vi "2013_01_03 Flow Motor.vi"(0 "Motor Typedef":T2={"Fail"=FALSE, "RPM"=0, "Motor"=enum."Maxon EC6 6V", "ESC"=enum."Phoenix 10", "Supply (V)"=0.0, "Elapsed Time"=0.0, "Counter"=0.0, "Torque (mNm)"=0.0, "Electrical Power (W)"=0.0, "Motor Efficiency"=0.0, "Mechanical Power (W)"=0.0, "Supply Power (W)"=0.0, "ESC Efficiency"=0.0, "PWM"=0, "Direction"=enum."Push"} {"PWM" min=0 max=100 step=1 scale=0.0..100.0; "ESC Efficiency" format="%#_3g%%"; "Supply Power (W)" format="%.3g"; "Mechanical Power (W)" format="%.3g"; "Motor Efficiency" format="%#_3g%%"; "Electrical Power (W)" format="%.3g"; "Torque (mNm)" format="%.3g"; "Elapsed Time" format="%<%H:%M:%S>t"; "Supply (V)" format="%.2f"; "RPM" scale=0.0..60000.0}, 1 "Motor Typedef 2":T2={"Fail"=FALSE, "RPM"=0, "Motor"=enum."Maxon EC6 6V", "ESC"=enum."Phoenix 10", "Supply (V)"=0.0, "Elapsed Time"=0.0, "Counter"=0.0, "Torque (mNm)"=0.0, "Electrical Power (W)"=0.0, "Motor Efficiency"=0.0, "Mechanical Power (W)"=0.0, "Supply Power (W)"=0.0, "ESC Efficiency"=0.0, "PWM"=0, "Direction"=enum."Push"} {"PWM" min=0 max=100 step=1 scale=0.0..100.0; "ESC Efficiency" format="%#_3g%%"; "Supply Power (W)" format="%.3g"; "Mechanical Power (W)" format="%.3g"; "Motor Efficiency" format="%#_3g%%"; "Electrical Power (W)" format="%.3g"; "Torque (mNm)" format="%.3g"; "Elapsed Time" format="%<%H:%M:%S>t"; "Supply (V)" format="%.2f"; "RPM" scale=0.0..60000.0}, 2 "Capture":bool, 5 "File Path":path, 6 "Zero":bool, 7 "Save":bool, 8 "Flow in":T1 {"Thermometer" scale=15.0..50.0; "Pressure Up (mmHg)" format="%#.1g"; "Pressure Down (mmHg)" format="%#.1g"; "Zero Up" format="%.2f"; "Hydraulic Power" scale=0.0..0.1 scale format="%#.2f"; "Flow" scale=0.0..8.0 scale format="%#.2f"; "Pressure Difference" scale=0.0..10.0 scale format="%#.2f"}, 9 "data":waveform(dbl)[](array[waveform]), 11 "File ID and Serial #s":string, 12 "DAQmx Task Name":refnum<k21>, 13 "Clear":bool, 14 "Comment":string) -> (3 "Motor Typedef Out 2":T2={"Fail"=FALSE, "RPM"=0, "Motor"=enum."Maxon EC6 6V", "ESC"=enum."Phoenix 10", "Supply (V)"=0.0, "Elapsed Time"=0.0, "Counter"=0.0, "Torque (mNm)"=0.0, "Electrical Power (W)"=0.0, "Motor Efficiency"=0.0, "Mechanical Power (W)"=0.0, "Supply Power (W)"=0.0, "ESC Efficiency"=0.0, "PWM"=0, "Direction"=enum."Push"} {"PWM" min=0 max=100 step=1 scale=0.0..100.0; "ESC Efficiency" format="%#_3g%%"; "Supply Power (W)" format="%.3g"; "Mechanical Power (W)" format="%.3g"; "Motor Efficiency" format="%#_3g%%"; "Electrical Power (W)" format="%.3g"; "Torque (mNm)" format="%.3g"; "Elapsed Time" format="%<%H:%M:%S>t"; "Supply (V)" format="%.2f"; "RPM" scale=0.0..60000.0}, 4 "Motor Typedef Out":T2={"Fail"=FALSE, "RPM"=0, "Motor"=enum."Maxon EC6 6V", "ESC"=enum."Phoenix 10", "Supply (V)"=0.0, "Elapsed Time"=0.0, "Counter"=0.0, "Torque (mNm)"=0.0, "Electrical Power (W)"=0.0, "Motor Efficiency"=0.0, "Mechanical Power (W)"=0.0, "Supply Power (W)"=0.0, "ESC Efficiency"=0.0, "PWM"=0, "Direction"=enum."Push"} {"PWM" min=0 max=100 step=1 scale=0.0..100.0; "ESC Efficiency" format="%#_3g%%"; "Supply Power (W)" format="%.3g"; "Mechanical Power (W)" format="%.3g"; "Motor Efficiency" format="%#_3g%%"; "Electrical Power (W)" format="%.3g"; "Torque (mNm)" format="%.3g"; "Elapsed Time" format="%<%H:%M:%S>t"; "Supply (V)" format="%.2f"; "RPM" scale=0.0..60000.0}, 10 "Flow and P out":T1 {"Thermometer" scale=15.0..50.0; "Pressure Up (mmHg)" format="%#.1g"; "Pressure Down (mmHg)" format="%#.1g"; "Zero Up" format="%.2f"; "Hydraulic Power" scale=0.0..0.1 scale format="%#.2f"; "Flow" scale=0.0..8.0 scale format="%#.2f"; "Pressure Difference" scale=0.0..10.0 scale format="%#.2f"}, 15 "Final Out":dynamicdata(graph))   [LabVIEW 2013]
uses:
  Flow Type Def.ctl
  flow and pressure.ctl
  <vilib>/measure/madcrms.llb/Basic Averaged DC-RMS for 1 Chan.vi
  <vilib>/express/express shared/transition.llb/Dynamic To Waveform Array.vi
  <vilib>/express/express signal manip/GetorSetDDTAttributes/Set DDT Attributes/SetT0.vi
  <vilib>/express/express shared/transition.llb/Waveform Array To Dynamic.vi
  <vilib>/express/express signal manip/GetorSetDDTAttributes/Set DDT Attributes/Set DDT Properties.xnode
  <vilib>/measure/NI_MAPro.lvlib
panel:
  in  "Motor 2 Enable":bool
  in  "error in (no error)":errorcluster
  out "error out":errorcluster
  out "Saving Data":bool
  # "Stopped"
  # "Stopped"
  # "Stopped"
  # "Stopped"
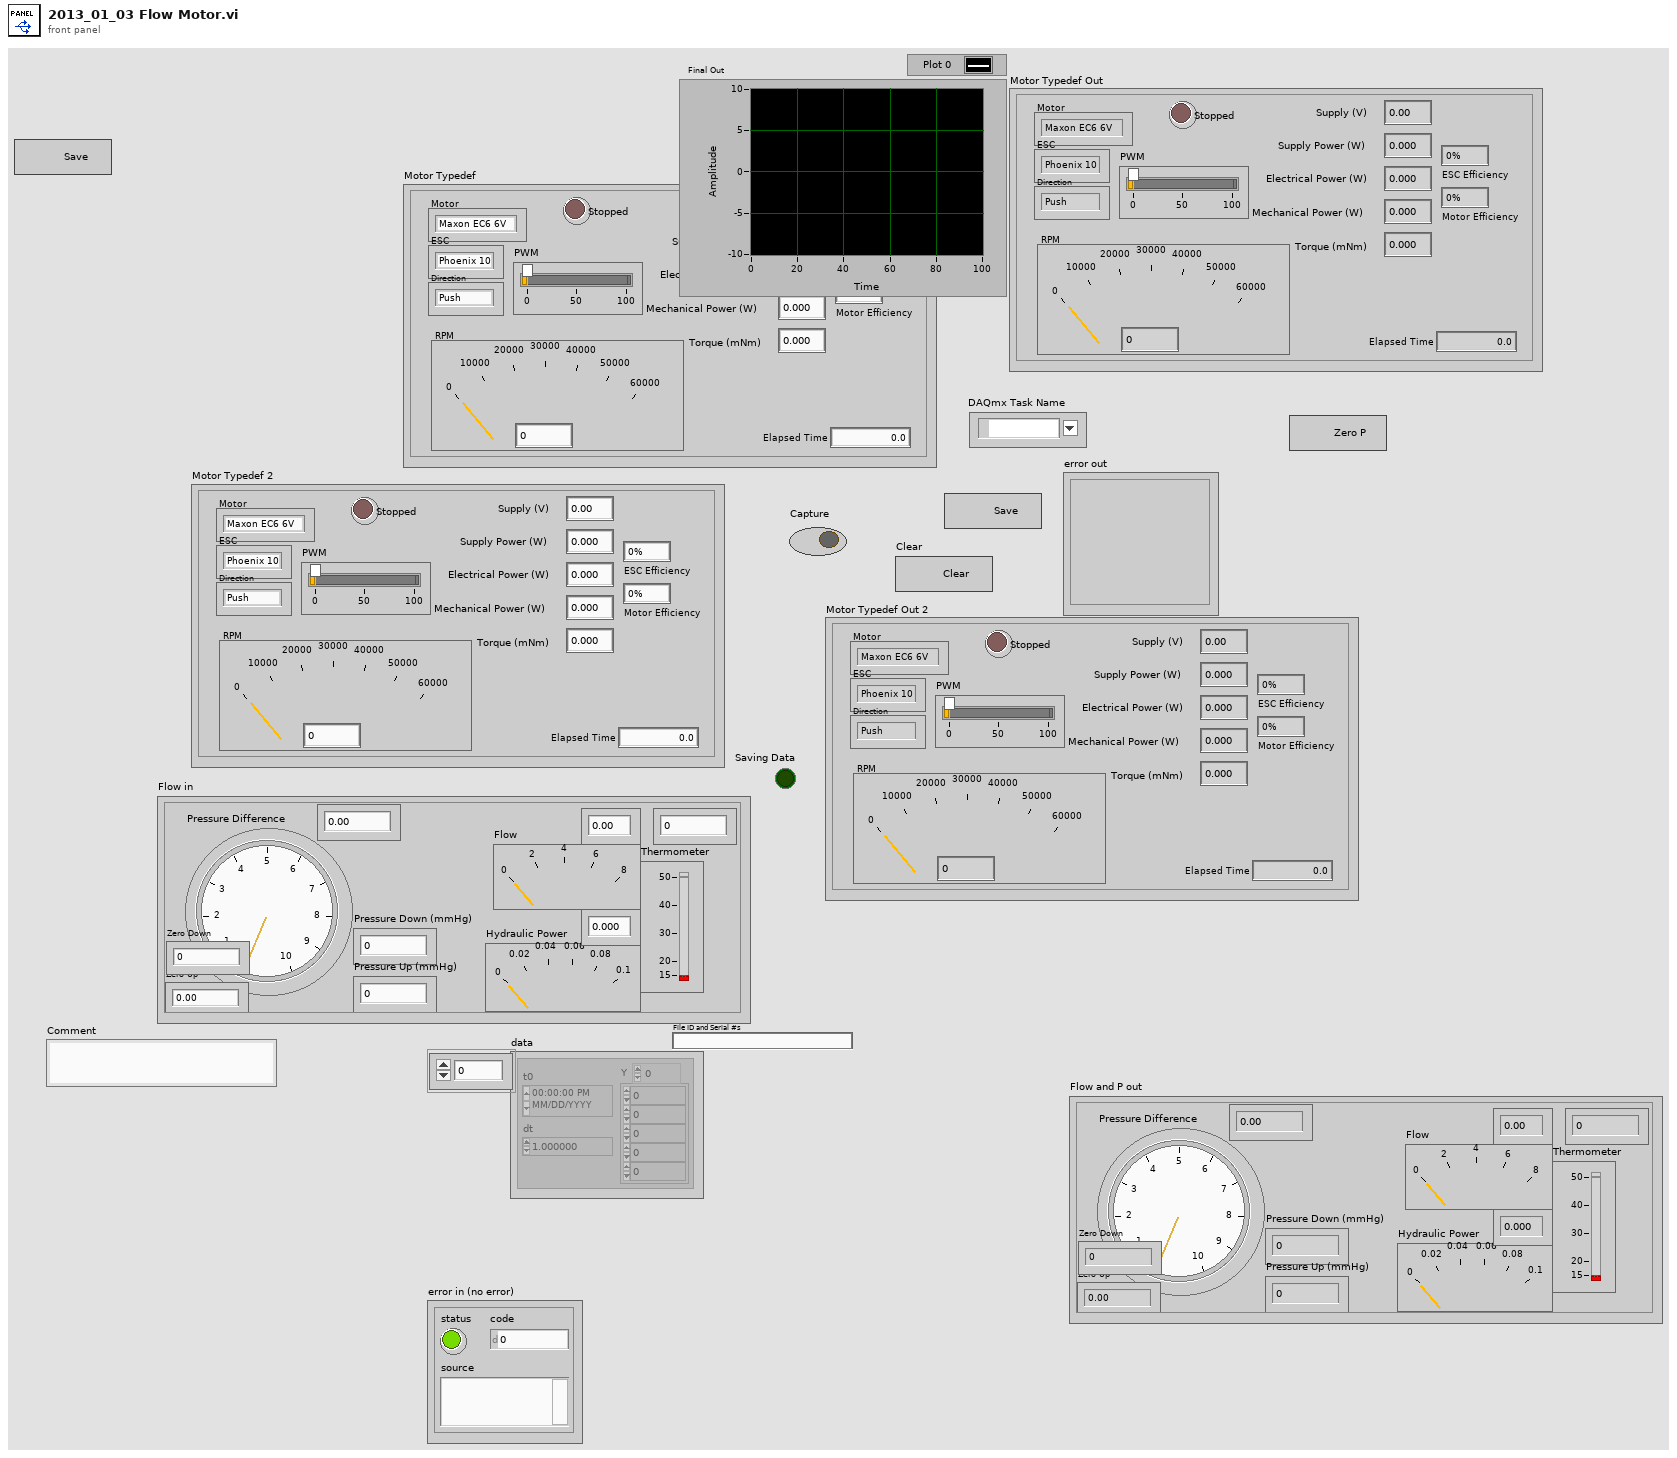
[diagram p1: front panel]
types:
  T1 = typedef "flow and pressure.ctl" = cluster{"Pressure Difference":dbl, "Flow":dbl, "Hydraulic Power":dbl, "Zero Up":dbl, "Pressure Down (mmHg)":dbl, "Pressure Up (mmHg)":dbl, "Zero Down":dbl, "Thermometer":dbl}
  T2 = typedef "Flow Type Def.ctl" = cluster{"Fail":bool, "RPM":u64, "Motor":enum16{"", "Maxon EC6 6V", "Maxon EC4 6V", "FH 0620 6V", "FH 0620 12V", "FH 0427"}, "ESC":enum16{"Phoenix 10", "Maxon", "FH 1801"}, "Supply (V)":dbl, "Elapsed Time":dbl, "Counter":dbl, "Torque (mNm)":dbl, "Electrical Power (W)":dbl, "Motor Efficiency":dbl, "Mechanical Power (W)":dbl, "Supply Power (W)":dbl, "ESC Efficiency":dbl, "PWM":i32, "Direction":enum16{"Push", "Pull"}}
  T3 = enum16{"", "Maxon EC6 6V", "Maxon EC4 6V", "FH 0620 6V", "FH 0620 12V", "FH 0427"}
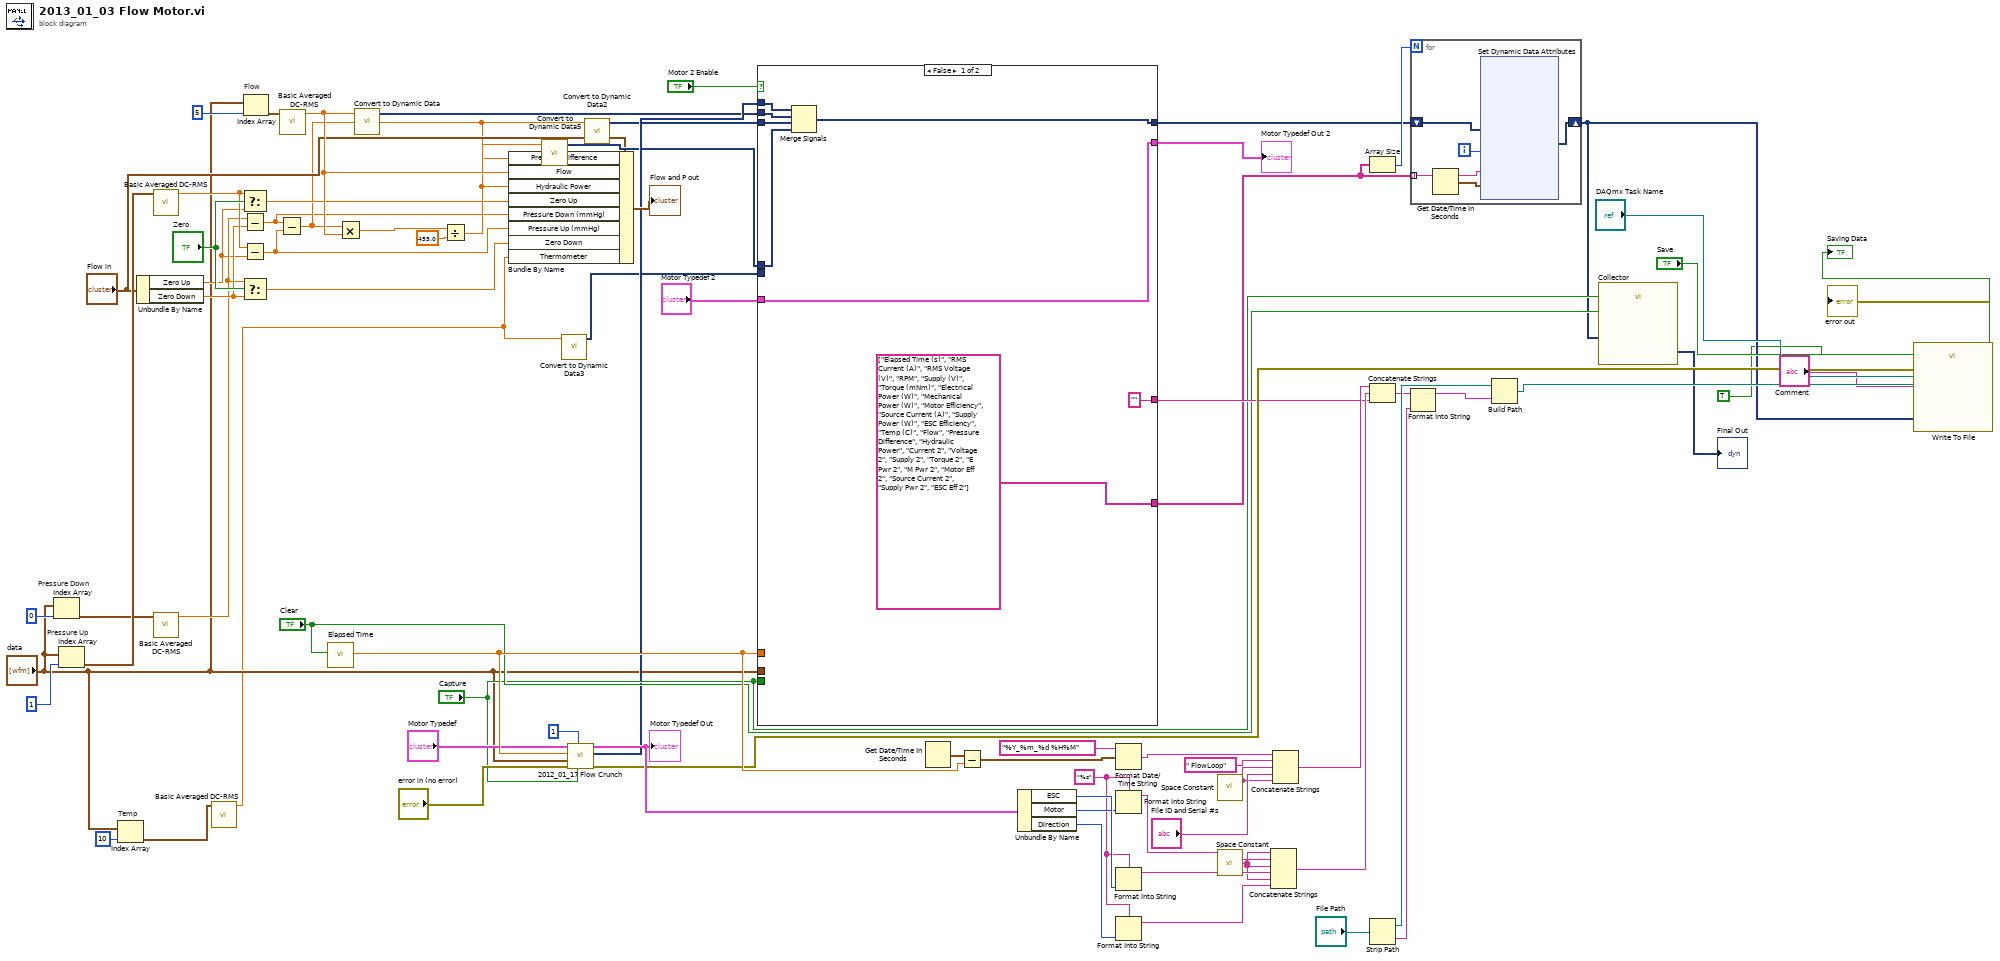
[diagram p0: block diagram]
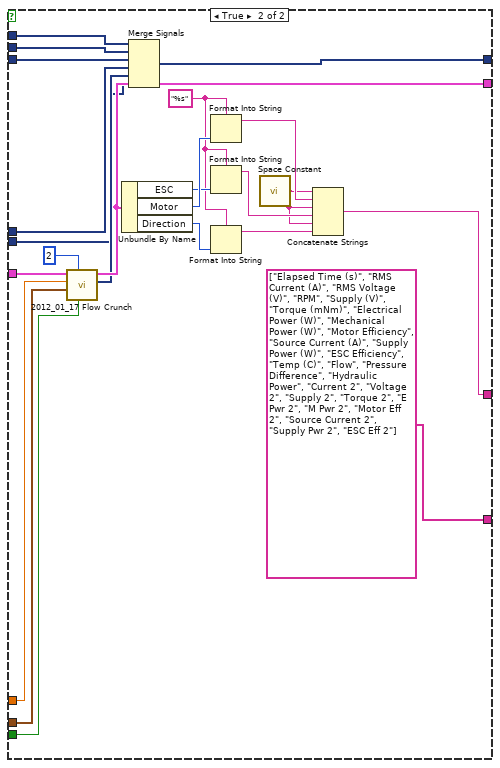
[diagram p2: hidden frame]
diagram:
  w30 = "%s" ("format string")
  n1 = Index Array "Pressure Down"(array="data", index=0) -> (element=w46:waveform(dbl))
  n2 = Index Array "Pressure Up"(array="data", index=1) -> (element=w47:waveform(dbl))
  n3 = Index Array "Temp"(array="data", index=10) -> (element=w5:waveform(dbl))
  n4 = Unbundle By Name("Flow in") -> ("Zero Up"=w10:dbl, "Zero Down"=w13:dbl)
  n5 = call-poly <vilib>:"Basic Averaged DC-RMS.vi"("signal in"=w47) -> ("DC value"=w14:dbl)  [unwired: 7 in, 3 out]
  n6 = call-poly <vilib>:"Basic Averaged DC-RMS.vi"("signal in"=w46) -> ("DC value"=w12:dbl)  [unwired: 7 in, 3 out]
  n7 = call-poly <vilib>:"Basic Averaged DC-RMS.vi"("signal in"=w5) -> ("DC value"=w4:dbl)  [unwired: 7 in, 3 out]
  n8 = Select(t=w14, s="Zero", f=w10) -> (s? t:f=w19:dbl)
  n9 = Subtract(x=w12, y=w13) -> (x-y=w9:dbl)
  n10 = Subtract(x=w14, y=w10) -> (x-y=w8:dbl)
  n11 = Select(t=w12, s="Zero", f=w13) -> (s? t:f=w15:dbl)
  n12 = Index Array "Flow"(array="data", index=5) -> (element=w48:waveform(dbl))
  n13 = Subtract(x=w9, y=w8) -> (x-y=w11:dbl)
  n14 = call-poly <vilib>:"Basic Averaged DC-RMS.vi"("signal in"=w48) -> ("DC value"=w41:dbl)  [unwired: 7 in, 3 out]
  n15 = call "Elapsed Time"("Reset"="Clear") -> ("Elapsed Time (s)"=w75:dbl)  [unwired: 11 in, 7 out]
  n16 = Multiply(x=w11, y=w41) -> (x*y=w40:dbl)
  n17 = call "Convert to Dynamic Data"("Double"=w41) -> ("Dynamic Data Type"=w24:dynamicdata)  [unwired: 3 in]
  n18 = Divide(x=w40, y=455.0) -> (x/y=w38:dbl)
  n19 = Bundle By Name(cluster="Flow in", "Pressure Difference"=w11, "Flow"=w41, "Hydraulic Power"=w38, "Zero Up"=w19, "Pressure Down (mmHg)"=w9, "Pressure Up (mmHg)"=w8, "Zero Down"=w15, "Thermometer"=w4) -> (→"Flow and P out":T1)
  n20 = call "Convert to Dynamic Data5"("Double"=w38) -> ("Dynamic Data Type"=w23:dynamicdata)  [unwired: 3 in]
  n21 = call "Convert to Dynamic Data3"("Double"=w4) -> ("Dynamic Data Type"=w3:dynamicdata)  [unwired: 3 in]
  n22 = call "2012_01_17 Flow Crunch.vi"("Capture"="Capture", "Motor #"=1, "error in (no error)"="error in (no error)", "data"="data", "Elapsed Time (s)"=w75, "Motor In"="Motor Typedef") -> ("error out"=w59:errorcluster, "Dynamic Data Type"=w25:dynamicdata, "Motor Out"=w73:T2)  [unwired: 3 in]
  "Motor Typedef Out" <- w73
  n23 = call "Convert to Dynamic Data2"("Double"=w11) -> ("Dynamic Data Type"=w18:dynamicdata)  [unwired: 3 in]
  n24 = case shown="False" "Motor 2 Enable" {
    tunnel: "data" -> [_ w108]
    tunnel: w75 -> [_ w107]
    tunnel: "Motor Typedef 2" -> [w85 w106]
    tunnel: [w85 w105] -> w70
    tunnel: ["" ("format string") w103] -> w49
    tunnel: "Capture" -> [_ w94]
    tunnel: w25 -> [w83 w93]
    tunnel: w24 -> [w82 w92]
    tunnel: w23 -> [w80 w88]
    tunnel: [string[] ["Elapsed Time (s)", "RMS Current (A)", "RMS Voltage (V)", "RPM", "Supply (V)", "Torque (mNm)", "Electrical Power (W)", "Mechanical Power (W)", "Motor Efficiency", "Source Current (A)", "Supply Power (W)", "ESC Efficiency", "Temp (C)", "Flow", "Pressure Difference", "Hydraulic Power", "Current 2", "Voltage 2", "Supply 2", "Torque 2", "E Pwr 2", "M Pwr 2", "Motor Eff 2", "Source Current 2", "Supply Pwr 2", "ESC Eff 2"] ("appended array") string[] ["Elapsed Time (s)", "RMS Current (A)", "RMS Voltage (V)", "RPM", "Supply (V)", "Torque (mNm)", "Electrical Power (W)", "Mechanical Power (W)", "Motor Efficiency", "Source Current (A)", "Supply Power (W)", "ESC Efficiency", "Temp (C)", "Flow", "Pressure Difference", "Hydraulic Power", "Current 2", "Voltage 2", "Supply 2", "Torque 2", "E Pwr 2", "M Pwr 2", "Motor Eff 2", "Source Current 2", "Supply Pwr 2", "ESC Eff 2"] ("appended array")] -> w22
    tunnel: [w81 w91] -> w21
    tunnel: w18 -> [w79 w89]
    tunnel: w3 -> [_ w86]
    frame False {
      n25 = Merge Signals(w83, w82, w79, w80) -> (w81:dynamicdata)
    }
    frame True {
      w96 = "%s" ("format string")
      n26 = call "2012_01_17 Flow Crunch.vi"("Capture"=w94, "Motor #"=2, "data"=w108, "Elapsed Time (s)"=w107, "Motor In"=w106) -> ("Dynamic Data Type"=w87:dynamicdata, "Motor Out"=w105:T2)  [unwired: 4 in, 1 out]
      n27 = Unbundle By Name(w105) -> ("ESC"=w100:enum16{"Phoenix 10", "Maxon", "FH 1801"}, "Motor"=w102:T3, "Direction"=w101:enum16{"Push", "Pull"})
      n28 = Merge Signals(w93, w92, w89, w88, w87, w86) -> (w91:dynamicdata)
      n29 = Format Into String(format string=w96, w102) -> (resulting string=w99:string)  [unwired: 2 in, 1 out]
      n30 = Format Into String(format string=w96, w100) -> (resulting string=w98:string)  [unwired: 2 in, 1 out]
      n31 = Format Into String(format string=w96, w101) -> (resulting string=w95:string)  [unwired: 2 in, 1 out]
      n32 = call <vilib>:"Space Constant.vi"() -> ("String"=w97:string)
      n33 = Concatenate Strings(w97, w99, w97, w98, w97, w95) -> (w103:string)
    }
  }
  "Motor Typedef Out 2" <- w70
  n34 = Get Date/Time In Seconds() -> (seconds since 1Jan1904=w63:timestamp)
  n35 = Subtract(x=w63, y=w75) -> (x-y=w62:timestamp)
  n36 = Unbundle By Name(w73) -> ("ESC"=w52:enum16{"Phoenix 10", "Maxon", "FH 1801"}, "Motor"=w51:T3, "Direction"=w50:enum16{"Push", "Pull"})
  n37 = Format Date/Time String(time format string (%c)="%Y_%m_%d %H%M", seconds (now)=w62) -> (date/time string=w58:string)  [unwired: 1 in]
  n38 = Format Into String(format string=w30, w51) -> (resulting string=w33:string)  [unwired: 2 in, 1 out]
  n39 = Format Into String(format string=w30, w52) -> (resulting string=w32:string)  [unwired: 2 in, 1 out]
  n40 = Format Into String(format string=w30, w50) -> (resulting string=w29:string)  [unwired: 2 in, 1 out]
  n41 = call <vilib>:"Space Constant.vi"() -> ("String"=w60:string)
  n42 = call <vilib>:"Space Constant.vi"() -> ("String"=w31:string)
  n43 = Concatenate Strings(w31, w33, w31, w32, w31, w29) -> (w54:string)
  n44 = Concatenate Strings(w58, " FlowLoop" ("string"), w60, "File ID and Serial #s", w60) -> (w55:string)
  n45 = Array Size(array=w22) -> (size(s)=w42:i32)
  n46 = Concatenate Strings(w55, w54, w49) -> (w53:string)
  n47 = Strip Path(path="File Path") -> (stripped path=w65:path, name=w66:string)
  n48 = for {
    N: w42 -> [_]
    tunnel: w22 -> [w111] mode=indexing
    shift-right: [w112] -> w17
    shift-left: w21 -> [w110]
    i -> [w113]
    n49 = Get Date/Time In Seconds() -> (seconds since 1Jan1904=w109:timestamp)
    n50 = xnode "Set Dynamic Data Attributes"("Signals In"=w110, "Signal Index"=w113, "Signal Name"=w111, "Timestamp"=w109) -> ("Signals Out"=w112:dynamicdata)  [unwired: 1 in, 1 out]
  }
  n51 = Format Into String(initial string=w53, w66) -> (resulting string=w64:string)  [unwired: 2 in, 1 out]
  n52 = Build Path(base path=w65, name or relative path=w64) -> (appended path=w67:path)
  n53 = call "Collector"("Reset"="Clear", "Enable"="Capture", "Signals"=w17) -> ("Collected Signals"=→"Final Out":dynamicdata)  [unwired: 7 in, 1 out]
  n54 = call "Write To File"("Signals"=w17, "Reset"=TRUE, "Enable"="Save", "error in (no error)"=w59, "Filename"=w67, "Comment"="Comment", "DAQmx Task"="DAQmx Task Name") -> ("Saving Data"=→"Saving Data":bool, "error out"=→"error out":errorcluster)  [unwired: 10 in, 1 out]
